vi "Split myDAQ DIO.vi"(2 "IN 7:0":u8 format="%08b") -> (5 "OUT 2, OUT0":fxp<+,2,2> format="%02b", 6 "OUT 1":bool, 7 "OUT 3":bool, 8 "OUT 7":bool, 9 "OUT 6, OUT 4":fxp<+,2,2> format="%02b", 10 "OUT 5":bool)   [LabVIEW 2013]
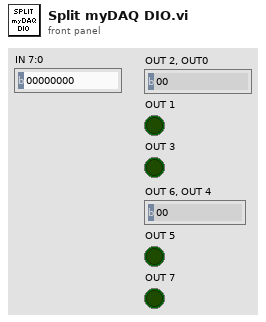
[diagram p1: front panel]
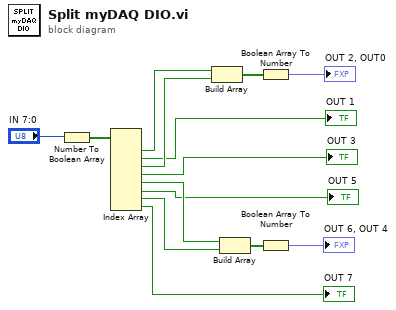
[diagram p0: block diagram]
diagram:
  n1 = Number To Boolean Array(number="IN 7:0") -> (Boolean array=w13:bool[])
  n2 = Index Array(array=w13) -> (element #1=w10:bool, element #2=→"OUT 1":bool, element #3=w9:bool, element #4=→"OUT 3":bool, element #5=w5:bool, element #6=→"OUT 5":bool, element #7=w4:bool, element #8=→"OUT 7":bool)  [unwired: 8 in]
  n3 = Build Array(w10, w9) -> (w7:bool[])
  n4 = Build Array(w5, w4) -> (w1:bool[])
  n5 = Boolean Array To Number(Boolean array=w7) -> (number=→"OUT 2, OUT0":fxp<+,2,2>)
  n6 = Boolean Array To Number(Boolean array=w1) -> (number=→"OUT 6, OUT 4":fxp<+,2,2>)
